vi "WORD.ReportGenerator.Title.vi"(8 "error in (no error)":errorcluster, 9 "Font":T1, 10 "Title":string, 11 "NI_report in":refnum<class "NI_report.lvclass">) -> (0 "error out":errorcluster, 3 "NI_report out":refnum<class "NI_report.lvclass">)   [LabVIEW 2019, in "Tools.lvlib"]
uses:
  <vilib>/Utility/NIReport.llb/NI_report.lvclass
  <vilib>/Utility/NIReport.llb/Append Report Text (str wrap).vi
  Tools.lvlib
  <vilib>/addons/_office/NI_ReportGenerationToolkit.lvlib
  <vilib>/Utility/NIReport.llb/Word/NI_Word.lvclass
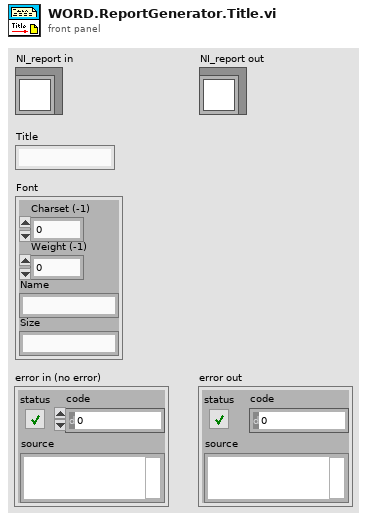
[diagram p1: front panel]
types:
  T1 = cluster{"Charset (-1)":i16, "Weight (-1)":i16, "Name":string, "Size":string}
  T2 = cluster{"Italic":enum16{"Italic Unchanged", "Italic On", "Italic Off"}, "Strike Through":enum16{"Strike Through Unchanged", "Strike Through On", "Strike Through Off"}, "Underline":enum16{"Underline Unchanged", "Underline On", "Underline Off"}, "Bold":enum16{"Bold Unchanged", "Bold On", "Bold Off"}}
  T3 = cluster{"Alignment":enum16{"Left", "Centered", "Right", "Justify"}, "Left":dbl, "Right":dbl, "Special":enum16{"(none)", "First line", "Hanging"}, "By":dbl, "Before":dbl, "After":dbl, "Line spacing":enum16{"Single", "1,5 lines", "Double", "At least", "Exactly", "Multiple"}, "At":dbl}
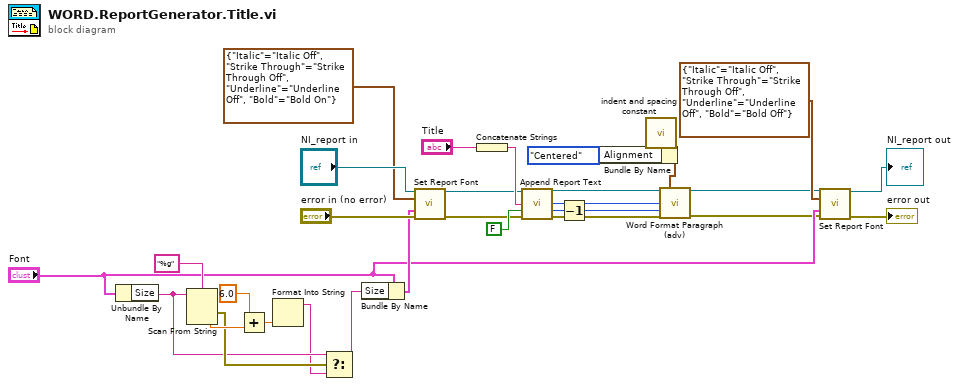
[diagram p0: block diagram]
diagram:
  n1 = Unbundle By Name("Font") -> ("Size"=w21:string)
  n2 = Scan From String(format string="%g", input string=w21) -> (error out=w22:errorcluster, output 1=w24:dbl)  [unwired: 3 in, 2 out]
  n3 = Add(x=6.0, y=w24) -> (x+y=w23:dbl)
  n4 = Format Into String(w23) -> (resulting string=w20:string)  [unwired: 3 in, 1 out]
  n5 = Select(t=w21, s=w22, f=w20) -> (s? t:f=w19:string)
  n6 = Bundle By Name(cluster="Font", "Size"=w19) -> (w18:T1)
  n7 = call-dynamic "Set Report Font.vi"("report in"="NI_report in", "text options"=T2 {"Italic"=enum."Italic Off", "Strike Through"=enum."Strike Through Off", "Underline"=enum."Underline Off", "Bold"=enum."Bold On"}, "font settings"=w18, "error in (no error)"="error in (no error)") -> ("report out"=w10:refnum<class "NI_report.lvclass">, "error out"=w9:errorcluster)  [unwired: 9 in, 1 out]
  n8 = Concatenate Strings("Title") -> (w16:string)
  n9 = call-poly <vilib>:"Append Report Text.vi"("report in"=w10, "text"=w16, "append on new line? (F)"=FALSE, "error in (no error)"=w9) -> ("report out"=w5:refnum<class "NI_report.lvclass">, "start out (Word)"=w7:i32, "end out (Word)"=w6:i32, "error out"=w8:errorcluster)  [unwired: 8 in]
  n10 = Decrement(x=w6) -> (x-1=w2:i32)
  n11 = call <vilib>:"indent and spacing constant.vi"() -> ("indent and spacing"=w13:T3)
  n12 = Bundle By Name(cluster=w13, "Alignment"=enum16{"Left", "Centered", "Right", "Justify"}."Centered") -> (w12:T3)
  n13 = call <vilib>:"Word Format Paragraph (adv).vi"("report in"=w5, "indent and spacing"=w12, "start (-1)"=w7, "end (-1)"=w2, "error in (no error)"=w8) -> ("report out"=w4:refnum<class "NI_report.lvclass">, "error out"=w3:errorcluster)  [unwired: 2 in, 7 out]
  n14 = call-dynamic "Set Report Font.vi"("report in"=w4, "text options"=T2 {"Italic"=enum."Italic Off", "Strike Through"=enum."Strike Through Off", "Underline"=enum."Underline Off", "Bold"=enum."Bold Off"}, "font settings"="Font", "error in (no error)"=w3) -> ("report out"=→"NI_report out":refnum<class "NI_report.lvclass">, "error out"=→"error out":errorcluster)  [unwired: 9 in, 1 out]
